vi "Teleop.vi"(10 "Match Info":T1={"Autonomous Elapsed Seconds"=0.0, "TeleOp Elapsed Seconds"=0.0, "Disabled Elapsed Seconds"=0.0, "Visited Autonomous"=FALSE, "Visited TeleOp"=FALSE, "Visited Disabled"=FALSE, "Autonomous Settings"={"Autonomous Style"=enum."Independent", "VI Refnum"=refnum}}, 11 "Call Context":T2) -> ()   [LabVIEW 2019]
doc: "This VI is called for each TeleOp packet received from the DS where the robot is not disabled. It is often used to read from the joysticks and update I/O or to update setpoints for timed control loops. It should complete and return within 20 milliseconds or it may miss DS packets."
uses:
  <vilib>/Rock Robotics/WPI/DriverStation/WPI_DriverStationDerivedRobotMode.ctl
  <vilib>/Rock Robotics/WPI/DriverStation/WPI_DriverStationMatch Info.ctl
  <vilib>/Rock Robotics/WPI/ThirdParty/JAS_Junk/TrajLib/Conv_Meters_Feet.vi
  <vilib>/Rock Robotics/WPI/ThirdParty/JAS_Junk/TrajLib/Conv_Radians_Deg.vi
  <vilib>/Rock Robotics/WPI/Utilities/WPI_GetSetVariantRefNum.vi
  <vilib>/Rock Robotics/Network Tables/NT Write Boolean Array.vi
  <vilib>/Rock Robotics/Network Tables/NT Write Numeric Array.vi
  Robot Global Data.vi
  <vilib>/Rock Robotics/Network Tables/NT Read Boolean.vi
  <vilib>/Rock Robotics/Network Tables/NT Read Number.vi
  <vilib>/Rock Robotics/WPI/ThirdParty/JAS_Junk/TrajLib/Trajectory_Library.lvlib
panel:
  out "Sample Slider 0":dbl(slide) scale=0.0..5.0
  out "Sample Boolean 1":bool
  out "Sample Boolean 0":bool
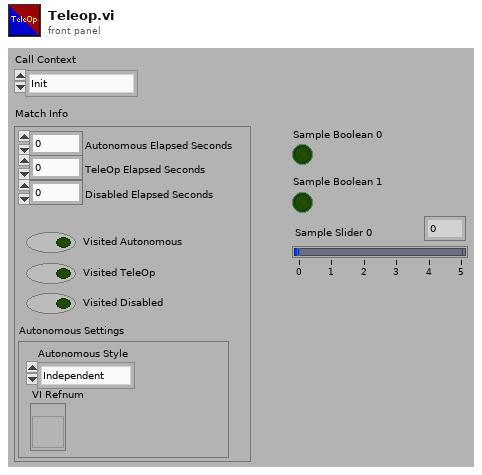
[diagram p1: front panel]
types:
  T1 = typedef "WPI_DriverStationMatch Info.ctl" = cluster{"Autonomous Elapsed Seconds":dbl, "TeleOp Elapsed Seconds":dbl, "Disabled Elapsed Seconds":dbl, "Visited Autonomous":bool, "Visited TeleOp":bool, "Visited Disabled":bool, "Autonomous Settings":cluster{"Autonomous Style":enum16{"Iterative", "Independent"}, "VI Refnum":refnum<vi>}}
  T2 = typedef "WPI_DriverStationDerivedRobotMode.ctl" = enum16{"Init", "Execute", "Stop"}
  T3 = typedef "WPI_JoystickDevRef.ctl" = cluster{"Device":T4}
  T4 = typedef "WPI_JoystickDeviceEnum.ctl" = enum16{"USB 0", "USB 1", "USB 2", "USB 3", "USB 4", "USB 5"}
  T5 = typedef "Trajectory_Library.lvlib/TRAJ_STATE.ctl" = cluster{"TimeSeconds":dbl, "Velocity":dbl, "Acceleration":dbl, "POSE":T6, "Curvature":dbl}
  T6 = typedef "Trajectory_Library.lvlib/POSE2D.ctl" = cluster{"TRANSLATION":T7, "ROTATION":T8}
  T7 = typedef "Trajectory_Library.lvlib/TRANSLATION2D.ctl" = cluster{"X":dbl, "Y":dbl}
  T8 = typedef "Trajectory_Library.lvlib/ROTATION2D.ctl" = cluster{"VALUE":dbl, "COS":dbl, "SIN":dbl}
  T9 = cluster{"Error Pose":T6, "X Corr":dbl, "Y Corr":dbl}
  T10 = typedef "Trajectory_Library.lvlib/CHASSIS_SPEEDS.ctl" = cluster{"vX":dbl, "vY":dbl, "vOmega":dbl}
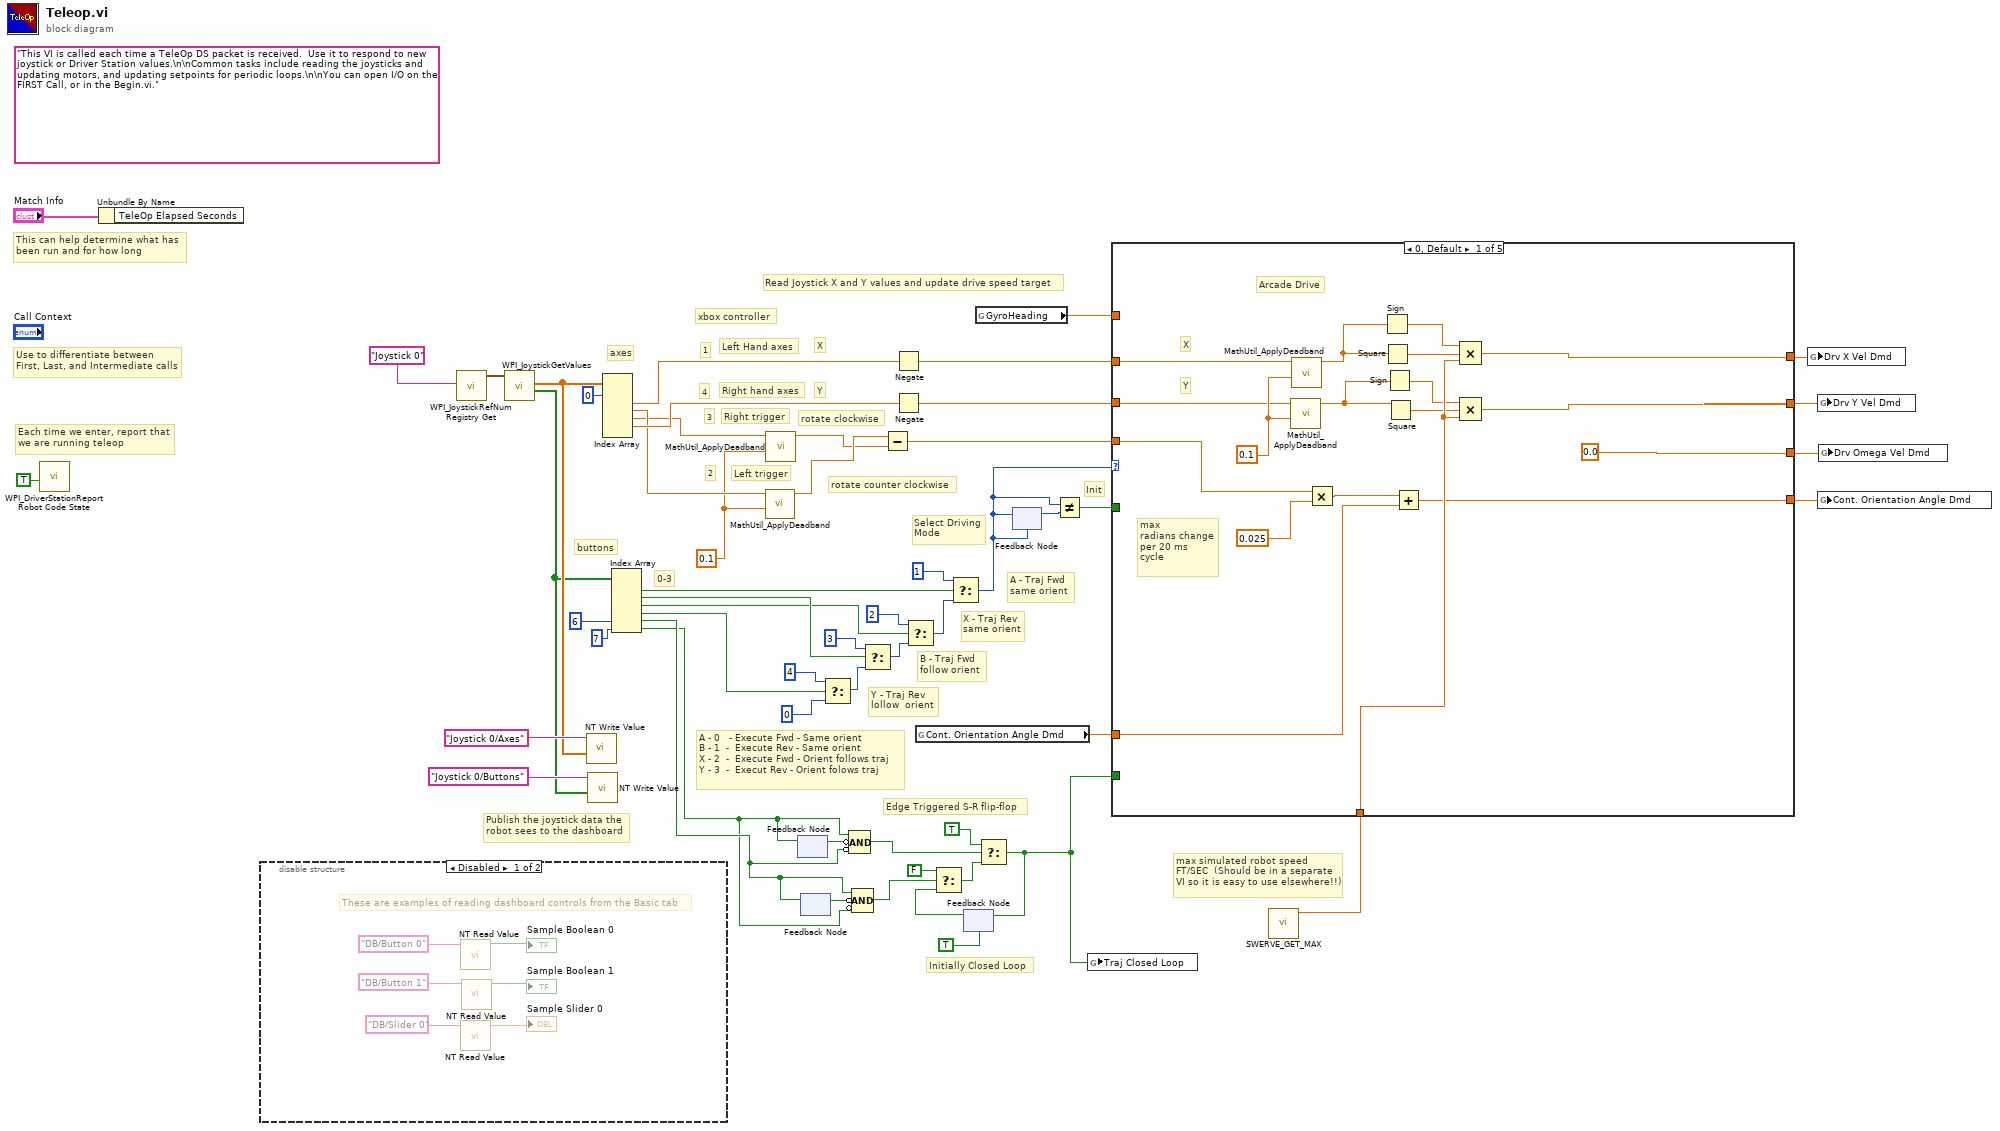
[diagram p0: block diagram]
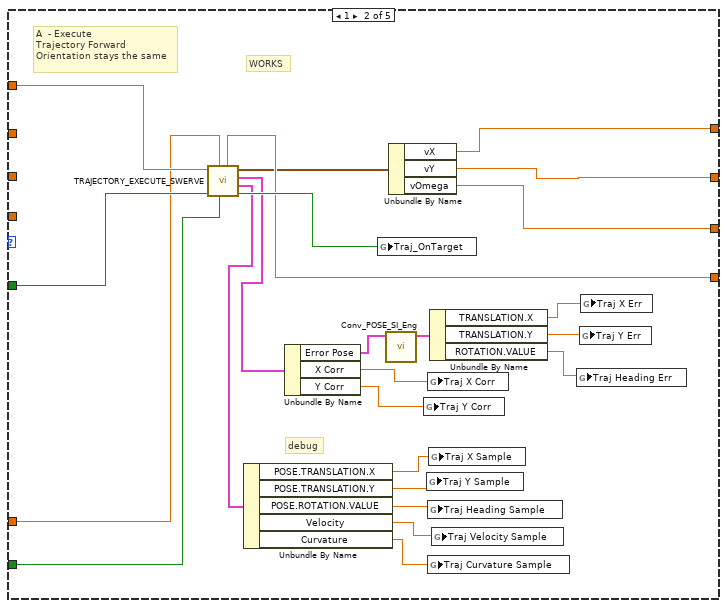
[diagram p2: hidden frame]
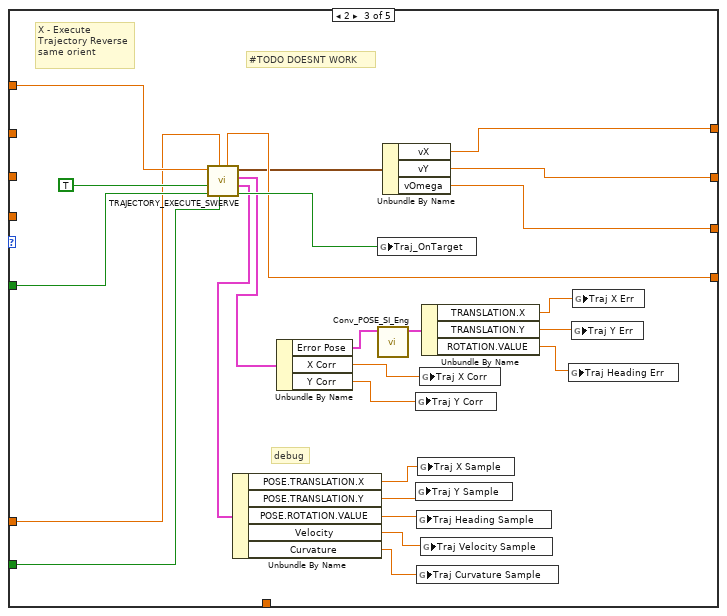
[diagram p3: hidden frame]
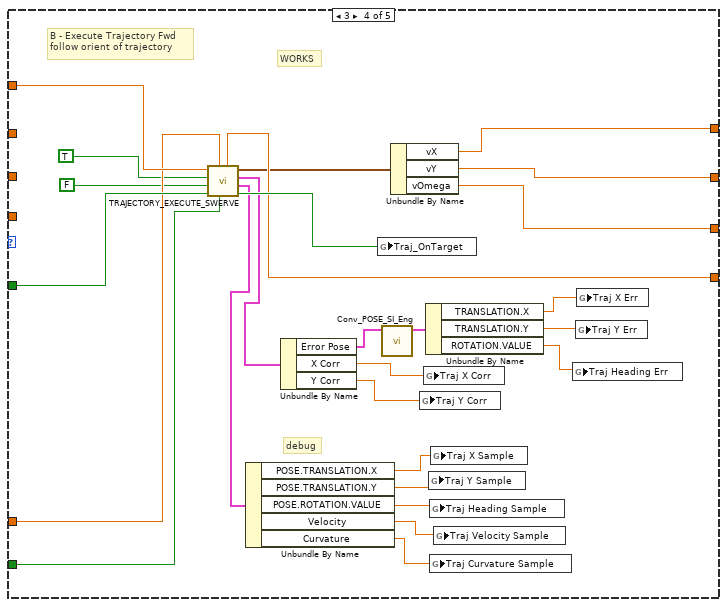
[diagram p4: hidden frame]
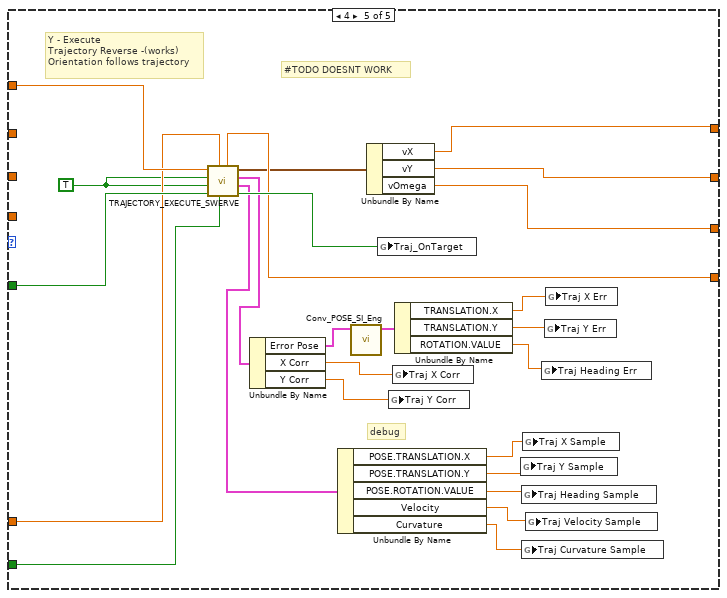
[diagram p5: hidden frame]
diagram:
  w3 = 0.1 ("Deadband")
  (unwired) "This VI is called each time a TeleOp DS packet is received.  Use it to respond to new joystick or Driver Station values.\n\nCommon tasks include reading the joysticks and updating motors, and updating setpoints for periodic loops.\n\nYou can open I/O on the FIRST Call, or in the Begin.vi."
  # "Edge Triggered S-R flip-flop"
  # "Initially Closed Loop"
  # "0-3"
  # "Init"
  # "Y - Traj Rev \nlollow  orient"
  # "B - Traj Fwd \nfollow orient"
  # "X - Traj Rev\nsame orient"
  # "A - 0   - Execute Fwd - Same orient\nB - 1  -  Execute Rev - Same orient\nX - 2  -  Execute Fwd - Orient follows traj\nY - 3  -  Execut Rev - Orient folows traj"
  # "A - Traj Fwd \nsame orient"
  # "xbox controller"
  # "Left trigger"
  # "rotate counter clockwise"
  # "2"
  # "Right trigger"
  # "rotate clockwise"
  # "3"
  # "Left Hand axes"
  # "1"
  # "4"
  # "Right hand axes"
  # "Y"
  # "X"
  # "Select Driving\nMode"
  # "buttons"
  # "axes"
  # "max simulated robot speed\nFT/SEC  (Should be in a separate\nVI so it is easy to use elsewhere!!)"
  # "Publish the joystick data the\nrobot sees to the dashboard"
  # "Each time we enter, report that\nwe are running teleop"
  # "Use to differentiate between\nFirst, Last, and Intermediate calls"
  # "This can help determine what has\nbeen run and for how long"
  # "Read Joystick X and Y values and update drive speed target"
  n1 = call <vilib>:"WPI_DriverStationReport Robot Code State.vi"("TeleOp"=TRUE ("Autonomous")) -> ()  [unwired: 10 in, 1 out]
  n2 = Unbundle By Name("Match Info") -> ()  [unwired: 1 out]
  n3 = disable-structure shown="Disabled" {
    frame Disabled {
      # "These are examples of reading dashboard controls from the Basic tab"
      n4 = call-poly <vilib>:"NT Read Value.vi"("Name"="DB/Button 0" ("refnum name")) -> ("Boolean"=→"Sample Boolean 0":bool)  [unwired: 9 in, 1 out]
      n5 = call-poly <vilib>:"NT Read Value.vi"("Name"="DB/Slider 0" ("refnum name")) -> ("Numeric"=→"Sample Slider 0":dbl)  [unwired: 9 in, 1 out]
      n6 = call-poly <vilib>:"NT Read Value.vi"("Name"="DB/Button 1" ("refnum name")) -> ("Boolean"=→"Sample Boolean 1":bool)  [unwired: 9 in, 1 out]
    }
    frame Enabled {
    }
  }
  n7 = call <vilib>:"WPI_JoystickRefNum Registry Get.vi"("refnum name"="Joystick 0") -> ("JoystickDevRef"=w53:T3)  [unwired: 1 in, 9 out]
  n8 = call <vilib>:"WPI_JoystickGetValues.vi"("JoystickDevRef"=w53) -> ("Buttons"=w46:bool[], "Axes"=w49:dbl[])  [unwired: 6 in, 3 out]
  n9 = call-poly <vilib>:"NT Write Value.vi"("Numeric Array"=w49, "Name"="Joystick 0/Axes") -> ()  [unwired: 9 in, 1 out]
  n10 = call-poly <vilib>:"NT Write Value.vi"("Boolean Array"=w46, "Name"="Joystick 0/Buttons") -> ()  [unwired: 9 in, 1 out]
  n11 = Index Array(array=w49, index #1=0 ("index")) -> (element #2=w29:dbl, element #3=w5:dbl, element #4=w2:dbl, element #5=w28:dbl)  [unwired: 5 in, 2 out]
  n12 = Index Array(array=w46, index #5=6 ("index"), index #6=7 ("index")) -> (element #1=w44:bool, element #2=w22:bool, element #3=w20:bool, element #4=w21:bool, element #5=w7:bool, element #6=w6:bool)  [unwired: 4 in]
  n13 = call <vilib>:"MathUtil_ApplyDeadband.vi"("Deadband"=w3, "Value"=w5) -> ("Result"=w4:dbl)  [unwired: 9 in]
  n14 = call <vilib>:"MathUtil_ApplyDeadband.vi"("Deadband"=w3, "Value"=w2) -> ("Result"=w1:dbl)  [unwired: 9 in]
  n15 = feedback-in #1(w6) -> ()
  n16 = feedback #1() -> (w17:bool)  [unwired: 1 in]
  n17 = feedback #2() -> (w16:bool)  [unwired: 1 in]
  n18 = feedback-in #2(w7) -> ()
  n19 = Select(t=4, s=w21, f=0) -> (s? t:f=w23:i32)
  n20 = Compound Arithmetic op=AND(w6, invert w17, invert w7) -> (w12:bool)
  n21 = Compound Arithmetic op=AND(w7, invert w16, invert w6) -> (w11:bool)
  n22 = Select(t=3, s=w22, f=w23) -> (s? t:f=w24:i32)
  n23 = Subtract(x=w4, y=w1) -> (x-y=w35:dbl)
  n24 = Negate(x=w29) -> (-x=w33:dbl)
  n25 = Negate(x=w28) -> (-x=w32:dbl)
  n26 = Select(t=2, s=w20, f=w24) -> (s? t:f=w30:i32)
  n27 = global read "Robot Global Data.vi" "Cont. Orientation Angle Dmd"() -> (w38:dbl)
  n28 = Select(t=1, s=w44, f=w30) -> (s? t:f=w42:i32)
  n29 = feedback #3(TRUE) -> (w10:bool)
  n30 = Select(t=FALSE, s=w11, f=w10) -> (s? t:f=w14:bool)
  n31 = global read "Robot Global Data.vi" "GyroHeading"() -> (w34:dbl)
  n32 = Select(t=TRUE, s=w12, f=w14) -> (s? t:f=w8:bool)
  n33 = feedback-in #3(w8) -> ()
  n34 = feedback-in #4(w42) -> ()
  n35 = feedback #4(w42) -> (w43:i32)
  n36 = Not Equal?(x=w42, y=w43) -> (x != y?=w41:bool)
  n37 = global write "Robot Global Data.vi" "Traj Closed Loop"(w8) -> ()
  n38 = call "SWERVE_GET_MAX.vi"() -> ("Max Wheel Vel (Meter/Sec)"=w40:dbl)  [unwired: 10 in, 1 out]
  n39 = case shown="0, Default" w42 {
    tunnel: w32 -> [w62 _ _ _ _]
    tunnel: [w79 w92 w116 w141 w163] -> w48
    tunnel: [w78 w91 w115 w140 w162] -> w47
    tunnel: w40 -> [w77 _ _ _ _]
    tunnel: w41 -> [_ w102 w127 w153 w174]
    tunnel: [w71 w99 w123 w150 w171] -> w39
    tunnel: w38 -> [w70 w100 w124 w151 w172]
    tunnel: [0.0 w90 w114 w139 w161] -> w37
    tunnel: w33 -> [w65 _ _ _ _]
    tunnel: w35 -> [w67 _ _ _ _]
    tunnel: w34 -> [_ w101 w126 w152 w173]
    tunnel: w8 -> [_ w88 w112 w137 w159]
    frame 0, Default {
      w63 = 0.1 ("Deadband")
      # "max \nradians change\nper 20 ms\ncycle"
      # "Y"
      # "X"
      # "Arcade Drive"
      n40 = call <vilib>:"MathUtil_ApplyDeadband.vi"("Deadband"=w63, "Value"=w62) -> ("Result"=w66:dbl)  [unwired: 9 in]
      n41 = call <vilib>:"MathUtil_ApplyDeadband.vi"("Deadband"=w63, "Value"=w65) -> ("Result"=w64:dbl)  [unwired: 9 in]
      n42 = Multiply(x=w67, y=0.025) -> (x*y=w69:dbl)
      n43 = Sign(1:w64) -> (0:w75:dbl)
      n44 = Square(x=w64) -> (x^2=w76:dbl)
      n45 = Sign(1:w66) -> (0:w73:dbl)
      n46 = Square(x=w66) -> (x^2=w74:dbl)
      n47 = Add(x=w69, y=w70) -> (x+y=w71:dbl)
      n48 = Compound Arithmetic op=MULTIPLY(w75, w76, w77) -> (w79:dbl)
      n49 = Compound Arithmetic op=MULTIPLY(w73, w74, w77) -> (w78:dbl)
    }
    frame 1 {
      # "debug"
      # "WORKS"
      # "A  - Execute\nTrajectory Forward\nOrientation stays the same"
      n50 = call "TRAJECTORY_EXECUTE_SWERVE.vi"("EnableClosedLoop"=w88, "Orientation Dmd In"=w100, "Init"=w102, "Gyro Heading"=w101) -> ("AtReference"=w103:bool, "OutputTRAJ_STATE"=w89:T5, "Error and Corr"=w80:T9, "Chassis Velocity Target"=w93:T10, "Orientation Target"=w99:dbl)  [unwired: 3 in]
      n51 = Unbundle By Name(w89) -> ("POSE.TRANSLATION.X"=w98:dbl, "POSE.TRANSLATION.Y"=w97:dbl, "POSE.ROTATION.VALUE"=w96:dbl, "Velocity"=w95:dbl, "Curvature"=w94:dbl)
      n52 = Unbundle By Name(w80) -> ("Error Pose"=w83:T6, "X Corr"=w82:dbl, "Y Corr"=w81:dbl)
      n53 = global write "Robot Global Data.vi" "Traj_OnTarget"(w103) -> ()
      n54 = call <vilib>:"Conv_POSE_SI_Eng.vi"("Err Pose in SI"=w83) -> ("Err Pose out ENG"=w87:T6)  [unwired: 10 in]
      n55 = Unbundle By Name(w93) -> ("vX"=w92:dbl, "vY"=w91:dbl, "vOmega"=w90:dbl)
      n56 = global write "Robot Global Data.vi" "Traj Y Corr"(w81) -> ()
      n57 = global write "Robot Global Data.vi" "Traj Y Sample"(w97) -> ()
      n58 = global write "Robot Global Data.vi" "Traj X Corr"(w82) -> ()
      n59 = global write "Robot Global Data.vi" "Traj Heading Sample"(w96) -> ()
      n60 = global write "Robot Global Data.vi" "Traj Curvature Sample"(w94) -> ()
      n61 = global write "Robot Global Data.vi" "Traj X Sample"(w98) -> ()
      n62 = Unbundle By Name(w87) -> ("TRANSLATION.X"=w86:dbl, "TRANSLATION.Y"=w85:dbl, "ROTATION.VALUE"=w84:dbl)
      n63 = global write "Robot Global Data.vi" "Traj Velocity Sample"(w95) -> ()
      n64 = global write "Robot Global Data.vi" "Traj Heading Err"(w84) -> ()
      n65 = global write "Robot Global Data.vi" "Traj Y Err"(w85) -> ()
      n66 = global write "Robot Global Data.vi" "Traj X Err"(w86) -> ()
    }
    frame 2 {
      # "debug"
      # "#TODO DOESNT WORK"
      # "X - Execute \nTrajectory Reverse\nsame orient"
      n67 = call "TRAJECTORY_EXECUTE_SWERVE.vi"("EnableClosedLoop"=w112, "Orientation Dmd In"=w124, "Init"=w127, "Reverse"=TRUE, "Gyro Heading"=w126) -> ("AtReference"=w128:bool, "OutputTRAJ_STATE"=w113:T5, "Error and Corr"=w104:T9, "Chassis Velocity Target"=w117:T10, "Orientation Target"=w123:dbl)  [unwired: 2 in]
      n68 = Unbundle By Name(w113) -> ("POSE.TRANSLATION.X"=w122:dbl, "POSE.TRANSLATION.Y"=w121:dbl, "POSE.ROTATION.VALUE"=w120:dbl, "Velocity"=w119:dbl, "Curvature"=w118:dbl)
      n69 = Unbundle By Name(w104) -> ("Error Pose"=w107:T6, "X Corr"=w106:dbl, "Y Corr"=w105:dbl)
      n70 = global write "Robot Global Data.vi" "Traj_OnTarget"(w128) -> ()
      n71 = call <vilib>:"Conv_POSE_SI_Eng.vi"("Err Pose in SI"=w107) -> ("Err Pose out ENG"=w111:T6)  [unwired: 10 in]
      n72 = Unbundle By Name(w117) -> ("vX"=w116:dbl, "vY"=w115:dbl, "vOmega"=w114:dbl)
      n73 = global write "Robot Global Data.vi" "Traj Y Corr"(w105) -> ()
      n74 = global write "Robot Global Data.vi" "Traj Y Sample"(w121) -> ()
      n75 = global write "Robot Global Data.vi" "Traj Heading Sample"(w120) -> ()
      n76 = global write "Robot Global Data.vi" "Traj Curvature Sample"(w118) -> ()
      n77 = global write "Robot Global Data.vi" "Traj X Sample"(w122) -> ()
      n78 = global write "Robot Global Data.vi" "Traj X Corr"(w106) -> ()
      n79 = global write "Robot Global Data.vi" "Traj Velocity Sample"(w119) -> ()
      n80 = Unbundle By Name(w111) -> ("TRANSLATION.X"=w110:dbl, "TRANSLATION.Y"=w109:dbl, "ROTATION.VALUE"=w108:dbl)
      n81 = global write "Robot Global Data.vi" "Traj Heading Err"(w108) -> ()
      n82 = global write "Robot Global Data.vi" "Traj Y Err"(w109) -> ()
      n83 = global write "Robot Global Data.vi" "Traj X Err"(w110) -> ()
    }
    frame 3 {
      # "debug"
      # "WORKS"
      # "B - Execute Trajectory Fwd \nfollow orient of trajectory"
      n84 = call "TRAJECTORY_EXECUTE_SWERVE.vi"("EnableClosedLoop"=w137, "Orientation Dmd In"=w151, "Init"=w153, "Reverse"=FALSE, "Follow Orientation"=TRUE ("Reverse"), "Gyro Heading"=w152) -> ("AtReference"=w154:bool, "OutputTRAJ_STATE"=w138:T5, "Error and Corr"=w129:T9, "Chassis Velocity Target"=w142:T10, "Orientation Target"=w150:dbl)  [unwired: 1 in]
      n85 = Unbundle By Name(w138) -> ("POSE.TRANSLATION.X"=w147:dbl, "POSE.TRANSLATION.Y"=w146:dbl, "POSE.ROTATION.VALUE"=w145:dbl, "Velocity"=w144:dbl, "Curvature"=w143:dbl)
      n86 = Unbundle By Name(w129) -> ("Error Pose"=w132:T6, "X Corr"=w131:dbl, "Y Corr"=w130:dbl)
      n87 = global write "Robot Global Data.vi" "Traj_OnTarget"(w154) -> ()
      n88 = call <vilib>:"Conv_POSE_SI_Eng.vi"("Err Pose in SI"=w132) -> ("Err Pose out ENG"=w136:T6)  [unwired: 10 in]
      n89 = Unbundle By Name(w142) -> ("vX"=w141:dbl, "vY"=w140:dbl, "vOmega"=w139:dbl)
      n90 = global write "Robot Global Data.vi" "Traj Y Corr"(w130) -> ()
      n91 = global write "Robot Global Data.vi" "Traj X Corr"(w131) -> ()
      n92 = Unbundle By Name(w136) -> ("TRANSLATION.X"=w135:dbl, "TRANSLATION.Y"=w134:dbl, "ROTATION.VALUE"=w133:dbl)
      n93 = global write "Robot Global Data.vi" "Traj Y Sample"(w146) -> ()
      n94 = global write "Robot Global Data.vi" "Traj Heading Sample"(w145) -> ()
      n95 = global write "Robot Global Data.vi" "Traj Curvature Sample"(w143) -> ()
      n96 = global write "Robot Global Data.vi" "Traj X Sample"(w147) -> ()
      n97 = global write "Robot Global Data.vi" "Traj Velocity Sample"(w144) -> ()
      n98 = global write "Robot Global Data.vi" "Traj Heading Err"(w133) -> ()
      n99 = global write "Robot Global Data.vi" "Traj Y Err"(w134) -> ()
      n100 = global write "Robot Global Data.vi" "Traj X Err"(w135) -> ()
    }
    frame 4 {
      w170 = TRUE ("Reverse")
      # "debug"
      # "#TODO DOESNT WORK"
      # "Y - Execute\nTrajectory Reverse -(works)\nOrientation follows trajectory"
      n101 = call "TRAJECTORY_EXECUTE_SWERVE.vi"("EnableClosedLoop"=w159, "Orientation Dmd In"=w172, "Init"=w174, "Reverse"=w170, "Follow Orientation"=w170, "Gyro Heading"=w173) -> ("AtReference"=w175:bool, "OutputTRAJ_STATE"=w160:T5, "Error and Corr"=w158:T9, "Chassis Velocity Target"=w164:T10, "Orientation Target"=w171:dbl)  [unwired: 1 in]
      n102 = Unbundle By Name(w158) -> ("Error Pose"=w157:T6, "X Corr"=w156:dbl, "Y Corr"=w155:dbl)
      n103 = Unbundle By Name(w160) -> ("POSE.TRANSLATION.X"=w169:dbl, "POSE.TRANSLATION.Y"=w168:dbl, "POSE.ROTATION.VALUE"=w167:dbl, "Velocity"=w166:dbl, "Curvature"=w165:dbl)
      n104 = call <vilib>:"Conv_POSE_SI_Eng.vi"("Err Pose in SI"=w157) -> ("Err Pose out ENG"=w179:T6)  [unwired: 10 in]
      n105 = Unbundle By Name(w164) -> ("vX"=w163:dbl, "vY"=w162:dbl, "vOmega"=w161:dbl)
      n106 = global write "Robot Global Data.vi" "Traj_OnTarget"(w175) -> ()
      n107 = global write "Robot Global Data.vi" "Traj Y Corr"(w155) -> ()
      n108 = global write "Robot Global Data.vi" "Traj X Corr"(w156) -> ()
      n109 = Unbundle By Name(w179) -> ("TRANSLATION.X"=w178:dbl, "TRANSLATION.Y"=w177:dbl, "ROTATION.VALUE"=w176:dbl)
      n110 = global write "Robot Global Data.vi" "Traj Y Sample"(w168) -> ()
      n111 = global write "Robot Global Data.vi" "Traj Heading Sample"(w167) -> ()
      n112 = global write "Robot Global Data.vi" "Traj Curvature Sample"(w165) -> ()
      n113 = global write "Robot Global Data.vi" "Traj X Sample"(w169) -> ()
      n114 = global write "Robot Global Data.vi" "Traj Velocity Sample"(w166) -> ()
      n115 = global write "Robot Global Data.vi" "Traj Heading Err"(w176) -> ()
      n116 = global write "Robot Global Data.vi" "Traj Y Err"(w177) -> ()
      n117 = global write "Robot Global Data.vi" "Traj X Err"(w178) -> ()
    }
  }
  n118 = global write "Robot Global Data.vi" "Drv X Vel Dmd"(w48) -> ()
  n119 = global write "Robot Global Data.vi" "Drv Y Vel Dmd"(w47) -> ()
  n120 = global write "Robot Global Data.vi" "Cont. Orientation Angle Dmd"(w39) -> ()
  n121 = global write "Robot Global Data.vi" "Drv Omega Vel Dmd"(w37) -> ()
